vi "Cmd-Rec New.vi"(4 "error in (no error)":errorcluster, 6 "recordset reference":T4, 7 "command reference":T5) -> (0 "error out":errorcluster, 3 "command-recordset reference":T2)   [LabVIEW 2012, in "NI_Database_API_64.lvlib"]
doc: "Creates and initializes a new <B>Command-Recordset</B> object.\n\nThis object should be destroyed using a <B>Command-Recordset Destroy</B> VI."
uses:
  NI_Database_API_64.lvlib
  Recordset.llb/Rec ObjectReference.ctl
  Command.llb/Cmd ObjectReference.ctl
  Cmd-Rec Data Members.ctl
  Cmd-Rec Object Reference.ctl
  <vilib>/Utility/_goopsup.llb/GOOP Object Repository Method.ctl
panel:
  in  "mode (create new)":T1(ring)
  out "status":enum16{"error", "new object", "existing object"}(ring)
  in  "command-recordset reference":T3
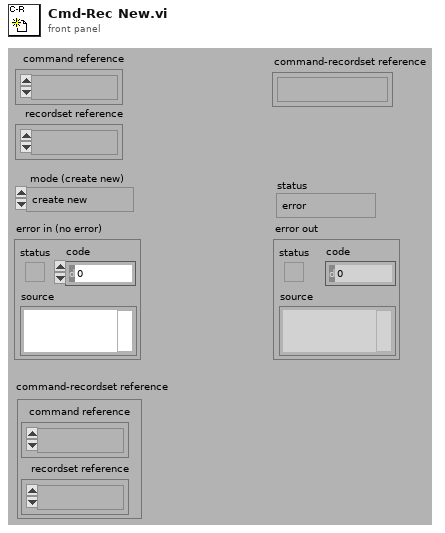
[diagram p1: front panel]
types:
  T1 = enum16{"create new", "lookup existing", "lookup or create"}
  T2 = typedef "NI_Database_API_64.lvlib/Cmd-Rec Object Reference.ctl" = refnum<k1>
  T3 = typedef "NI_Database_API_64.lvlib/Cmd-Rec Data Members.ctl" = cluster{"recordset reference":T4, "command reference":T5}
  T4 = typedef "NI_Database_API_64.lvlib/Rec ObjectReference.ctl" = refnum<k1>
  T5 = typedef "NI_Database_API_64.lvlib/Cmd ObjectReference.ctl" = refnum<k1>
  T6 = typedef "GOOP Object Repository Method.ctl" = enum16{"Create", "GetCopy", "GetModify", "Set", "Destroy", "Create Static", "Get All Refs", "Reset", "Get Statistics"}
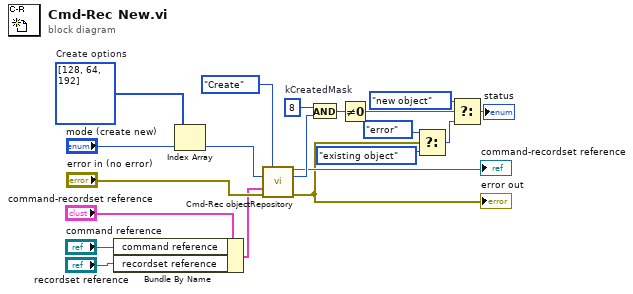
[diagram p0: block diagram]
diagram:
  w6 = 8  # kCreatedMask
  w9 = i32[] [128, 64, 192]  # Create options
  n1 = Bundle By Name(cluster="command-recordset reference", "command reference"="command reference", "recordset reference"="recordset reference") -> (w1:T3)
  n2 = Index Array(array=w9, index="mode (create new)") -> (element=w10:i32)
  n3 = call "Cmd-Rec objectRepository.vi"("method"=GOOP_Object_Repository_Method."Create", "flags in"=w10, "classDataIn"=w1, "error in (no error)"="error in (no error)") -> ("command-recordset reference out"=→"command-recordset reference":T2, "flags out"=w7:i32, "error out"=w2:errorcluster)  [unwired: 5 in, 4 out]
  "error out" <- w2
  n4 = And(x=w6, y=w7) -> (x .and. y?=w11:i32)
  n5 = Not Equal To 0?(x=w11) -> (x != 0?=w12:bool)
  n6 = Select(t=enum16{"error", "new object", "existing object"}."error" ("status"), s=w2, f=enum16{"error", "new object", "existing object"}."existing object" ("status")) -> (s? t:f=w16:enum16{"error", "new object", "existing object"})
  n7 = Select(t=enum16{"error", "new object", "existing object"}."new object" ("status"), s=w12, f=w16) -> (s? t:f=→"status":enum16{"error", "new object", "existing object"})
